vi "Autonomous.vi"   [LabVIEW 2017]
doc: "This VI starts when autonomous period begins, and will automatically be terminated when it ends. You can carry out timed or sensor driven operations directly to I/O or to subsystems without needing to return to the caller."
uses:
  <vilib>/Rock Robotics/WPI/Utilities/WPI_GetSetVariantRefNum.vi
  <vilib>/Rock Robotics/Network Tables/NT Read String.vi
types:
  T1 = typedef "WPI_JoystickDevRef.ctl" = cluster{"Device":T2}
  T2 = typedef "WPI_JoystickDeviceEnum.ctl" = enum16{"USB 0", "USB 1", "USB 2", "USB 3", "USB 4", "USB 5"}
  T3 = typedef "Command Status Info.ctl" = cluster{"Name":string, "Status":T4, "notifier out":T5}
  T4 = typedef "Completion Status.ctl" = enum16{"Successful", "Aborted", "Incomplete"}
  T5 = typedef "Completion Notifier.ctl" = refnum<notifier>
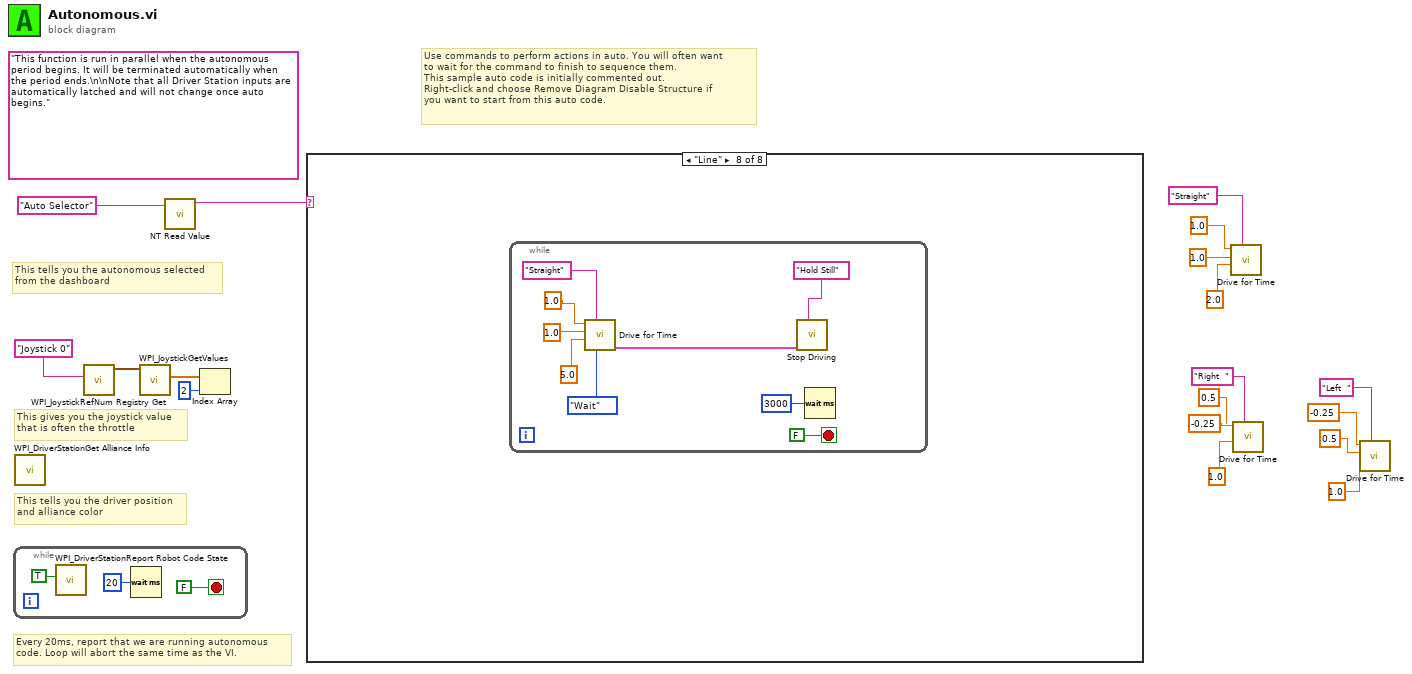
[diagram p0: block diagram]
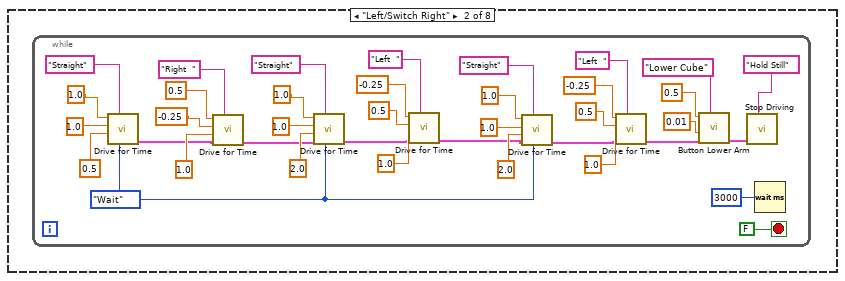
[diagram p3: hidden frame]
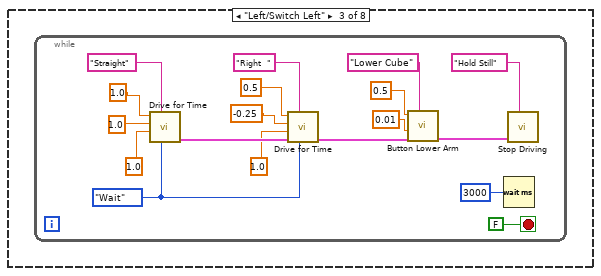
[diagram p4: hidden frame]
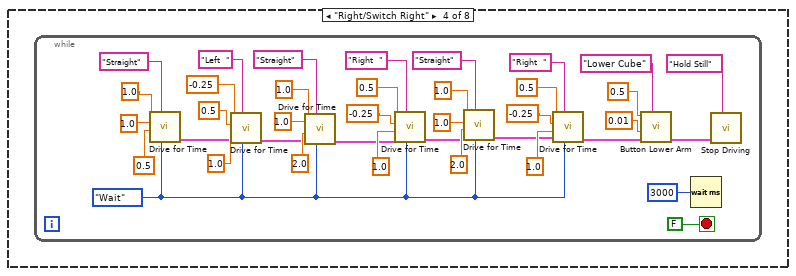
[diagram p5: hidden frame]
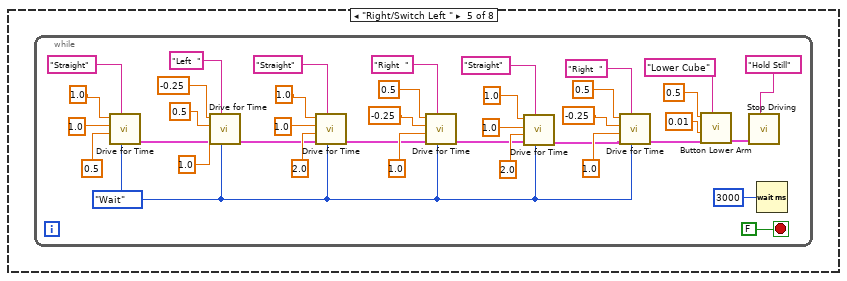
[diagram p6: hidden frame]
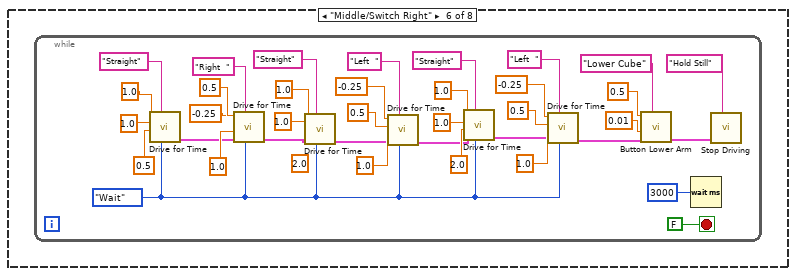
[diagram p7: hidden frame]
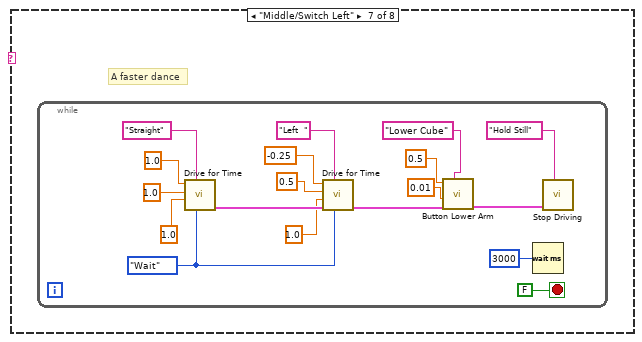
[diagram p8: hidden frame]
diagram:
  (unwired) "This function is run in parallel when the autonomous period begins. It will be terminated automatically when the period ends.\n\nNote that all Driver Station inputs are automatically latched and will not change once auto begins."
  # "Use commands to perform actions in auto. You will often want\nto wait for the command to finish to sequence them.\nThis sample auto code is initially commented out. \nRight-click and choose Remove Diagram Disable Structure if\nyou want to start from this auto code."
  # "This tells you the autonomous selected\nfrom the dashboard"
  # "Every 20ms, report that we are running autonomous\ncode. Loop will abort the same time as the VI."
  # "This gives you the joystick value\nthat is often the throttle"
  # "This tells you the driver position\nand alliance color"
  n1 = while {
    stop <- FALSE stop-if-true
    n2 = call <vilib>:"WPI_DriverStationReport Robot Code State.vi"("Autonomous"=TRUE) -> ()  [unwired: 10 in, 1 out]
    n3 = Wait (ms)(milliseconds to wait=u32 20) -> ()  [unwired: 1 out]
  }
  n4 = call <vilib>:"WPI_DriverStationGet Alliance Info.vi"() -> ()  [unwired: 12 out]
  n5 = call <vilib>:"WPI_JoystickRefNum Registry Get.vi"("refnum name"="Joystick 0") -> ("JoystickDevRef"=w17:T1)  [unwired: 1 in, 9 out]
  n6 = call <vilib>:"WPI_JoystickGetValues.vi"("JoystickDevRef"=w17) -> ("Axes"=w16:dbl[])  [unwired: 6 in, 4 out]
  n7 = call-poly <vilib>:"NT Read Value.vi"("Name"="Auto Selector") -> ("String"=w13:string)  [unwired: 9 in, 1 out]
  n8 = Index Array(array=w16, index=2) -> ()  [unwired: 1 out]
  n9 = case shown="\"Line\"" w13 {
    frame Default {
    }
    frame "Left/Switch Right" {
      n10 = while {
        stop <- FALSE stop-if-true
        w40 = enum16{"Start", "Wait"}."Wait" ("Synchronication")
        n11 = call "Drive for Time.vi"("Synchronization"=w40, "Description"="Straight", "Seconds"=0.5 ("Delay (s)"), "Right Speed"=1.0 ("X axis value"), "Left Speed"=1.0 ("X axis value")) -> ("Command Info Out"=w35:T3)  [unwired: 5 in, 1 out]
        n12 = call "Drive for Time.vi"("Description"="Right  ", "Command Info In"=w35, "Seconds"=1.0 ("Delay (s)"), "Right Speed"=-0.25 ("X axis value"), "Left Speed"=0.5 ("X axis value")) -> ("Command Info Out"=w34:T3)  [unwired: 5 in, 1 out]
        n13 = call "Drive for Time.vi"("Synchronization"=w40, "Description"="Straight", "Command Info In"=w34, "Seconds"=2.0 ("Delay (s)"), "Right Speed"=1.0 ("X axis value"), "Left Speed"=1.0 ("X axis value")) -> ("Command Info Out"=w29:T3)  [unwired: 4 in, 1 out]
        n14 = call "Drive for Time.vi"("Description"="Left  ", "Command Info In"=w29, "Seconds"=1.0 ("Delay (s)"), "Right Speed"=0.5 ("X axis value"), "Left Speed"=-0.25 ("X axis value")) -> ("Command Info Out"=w28:T3)  [unwired: 5 in, 1 out]
        n15 = call "Drive for Time.vi"("Synchronization"=w40, "Description"="Straight", "Command Info In"=w28, "Seconds"=2.0 ("Delay (s)"), "Right Speed"=1.0 ("X axis value"), "Left Speed"=1.0 ("X axis value")) -> ("Command Info Out"=w23:T3)  [unwired: 4 in, 1 out]
        n16 = call "Drive for Time.vi"("Description"="Left  ", "Command Info In"=w23, "Seconds"=1.0 ("Delay (s)"), "Right Speed"=0.5 ("X axis value"), "Left Speed"=-0.25 ("X axis value")) -> ("Command Info Out"=w22:T3)  [unwired: 5 in, 1 out]
        n17 = call "Button Lower Arm.vi"("Description"="Lower Cube", "Command Info In"=w22, "Deadband Value"=0.01, "Setpoint"=0.5) -> ("Command Info Out"=w57:T3)  [unwired: 7 in]
        n18 = call "Stop Driving.vi"("Description"="Hold Still", "Command Info In"=w57) -> ()  [unwired: 9 in, 1 out]
        n19 = Wait (ms)(milliseconds to wait=u32 3000 ("millisecond timer value")) -> ()  [unwired: 1 out]
      }
    }
    frame "Left/Switch Left" {
      n20 = while {
        stop <- FALSE stop-if-true
        w65 = enum16{"Start", "Wait"}."Wait" ("Synchronication")
        n21 = call "Drive for Time.vi"("Synchronization"=w65, "Description"="Straight", "Seconds"=1.0 ("Delay (s)"), "Right Speed"=1.0 ("X axis value"), "Left Speed"=1.0 ("X axis value")) -> ("Command Info Out"=w77:T3)  [unwired: 5 in, 1 out]
        n22 = call "Drive for Time.vi"("Synchronization"=w65, "Description"="Right  ", "Command Info In"=w77, "Seconds"=1.0 ("Delay (s)"), "Right Speed"=-0.25 ("X axis value"), "Left Speed"=0.5 ("X axis value")) -> ("Command Info Out"=w62:T3)  [unwired: 4 in, 1 out]
        n23 = call "Button Lower Arm.vi"("Description"="Lower Cube", "Command Info In"=w62, "Deadband Value"=0.01, "Setpoint"=0.5) -> ("Command Info Out"=w60:T3)  [unwired: 7 in]
        n24 = Wait (ms)(milliseconds to wait=u32 3000 ("millisecond timer value")) -> ()  [unwired: 1 out]
        n25 = call "Stop Driving.vi"("Description"="Hold Still", "Command Info In"=w60) -> ()  [unwired: 9 in, 1 out]
      }
    }
    frame "Right/Switch Right" {
      n26 = while {
        stop <- FALSE stop-if-true
        w78 = enum16{"Start", "Wait"}."Wait" ("Synchronication")
        n27 = call "Drive for Time.vi"("Synchronization"=w78, "Description"="Straight", "Seconds"=0.5 ("Delay (s)"), "Right Speed"=1.0 ("X axis value"), "Left Speed"=1.0 ("X axis value")) -> ("Command Info Out"=w95:T3)  [unwired: 5 in, 1 out]
        n28 = call "Drive for Time.vi"("Synchronization"=w78, "Description"="Left  ", "Command Info In"=w95, "Seconds"=1.0 ("Delay (s)"), "Right Speed"=0.5 ("X axis value"), "Left Speed"=-0.25 ("X axis value")) -> ("Command Info Out"=w90:T3)  [unwired: 4 in, 1 out]
        n29 = call "Drive for Time.vi"("Synchronization"=w78, "Description"="Straight", "Command Info In"=w90, "Seconds"=2.0 ("Delay (s)"), "Right Speed"=1.0 ("X axis value"), "Left Speed"=1.0 ("X axis value")) -> ("Command Info Out"=w85:T3)  [unwired: 4 in, 1 out]
        n30 = call "Drive for Time.vi"("Synchronization"=w78, "Description"="Right  ", "Command Info In"=w85, "Seconds"=1.0 ("Delay (s)"), "Right Speed"=-0.25 ("X axis value"), "Left Speed"=0.5 ("X axis value")) -> ("Command Info Out"=w80:T3)  [unwired: 4 in, 1 out]
        n31 = call "Drive for Time.vi"("Synchronization"=w78, "Description"="Straight", "Command Info In"=w80, "Seconds"=2.0 ("Delay (s)"), "Right Speed"=1.0 ("X axis value"), "Left Speed"=1.0 ("X axis value")) -> ("Command Info Out"=w79:T3)  [unwired: 4 in, 1 out]
        n32 = call "Drive for Time.vi"("Synchronization"=w78, "Description"="Right  ", "Command Info In"=w79, "Seconds"=1.0 ("Delay (s)"), "Right Speed"=-0.25 ("X axis value"), "Left Speed"=0.5 ("X axis value")) -> ("Command Info Out"=w102:T3)  [unwired: 4 in, 1 out]
        n33 = call "Button Lower Arm.vi"("Description"="Lower Cube", "Command Info In"=w102, "Deadband Value"=0.01, "Setpoint"=0.5) -> ("Command Info Out"=w100:T3)  [unwired: 7 in]
        n34 = Wait (ms)(milliseconds to wait=u32 3000 ("millisecond timer value")) -> ()  [unwired: 1 out]
        n35 = call "Stop Driving.vi"("Description"="Hold Still", "Command Info In"=w100) -> ()  [unwired: 9 in, 1 out]
      }
    }
    frame "Right/Switch Left " {
      n36 = while {
        stop <- FALSE stop-if-true
        w116 = enum16{"Start", "Wait"}."Wait" ("Synchronication")
        n37 = call "Drive for Time.vi"("Synchronization"=w116, "Description"="Straight", "Seconds"=0.5 ("Delay (s)"), "Right Speed"=1.0 ("X axis value"), "Left Speed"=1.0 ("X axis value")) -> ("Command Info Out"=w134:T3)  [unwired: 5 in, 1 out]
        n38 = call "Drive for Time.vi"("Synchronization"=w116, "Description"="Left  ", "Command Info In"=w134, "Seconds"=1.0 ("Delay (s)"), "Right Speed"=0.5 ("X axis value"), "Left Speed"=-0.25 ("X axis value")) -> ("Command Info Out"=w129:T3)  [unwired: 4 in, 1 out]
        n39 = call "Drive for Time.vi"("Synchronization"=w116, "Description"="Straight", "Command Info In"=w129, "Seconds"=2.0 ("Delay (s)"), "Right Speed"=1.0 ("X axis value"), "Left Speed"=1.0 ("X axis value")) -> ("Command Info Out"=w128:T3)  [unwired: 4 in, 1 out]
        n40 = call "Drive for Time.vi"("Synchronization"=w116, "Description"="Right  ", "Command Info In"=w128, "Seconds"=1.0 ("Delay (s)"), "Right Speed"=-0.25 ("X axis value"), "Left Speed"=0.5 ("X axis value")) -> ("Command Info Out"=w123:T3)  [unwired: 4 in, 1 out]
        n41 = call "Drive for Time.vi"("Synchronization"=w116, "Description"="Straight", "Command Info In"=w123, "Seconds"=2.0 ("Delay (s)"), "Right Speed"=1.0 ("X axis value"), "Left Speed"=1.0 ("X axis value")) -> ("Command Info Out"=w118:T3)  [unwired: 4 in, 1 out]
        n42 = call "Drive for Time.vi"("Synchronization"=w116, "Description"="Right  ", "Command Info In"=w118, "Seconds"=1.0 ("Delay (s)"), "Right Speed"=-0.25 ("X axis value"), "Left Speed"=0.5 ("X axis value")) -> ("Command Info Out"=w117:T3)  [unwired: 4 in, 1 out]
        n43 = call "Button Lower Arm.vi"("Description"="Lower Cube", "Command Info In"=w117, "Deadband Value"=0.01, "Setpoint"=0.5) -> ("Command Info Out"=w151:T3)  [unwired: 7 in]
        n44 = call "Stop Driving.vi"("Description"="Hold Still", "Command Info In"=w151) -> ()  [unwired: 9 in, 1 out]
        n45 = Wait (ms)(milliseconds to wait=u32 3000 ("millisecond timer value")) -> ()  [unwired: 1 out]
      }
    }
    frame "Middle/Switch Right" {
      n46 = while {
        stop <- FALSE stop-if-true
        (unwired) 2.0 ("Delay (s)")
        w154 = enum16{"Start", "Wait"}."Wait" ("Synchronication")
        n47 = call "Drive for Time.vi"("Synchronization"=w154, "Description"="Straight", "Seconds"=0.5 ("Delay (s)"), "Right Speed"=1.0 ("X axis value"), "Left Speed"=1.0 ("X axis value")) -> ("Command Info Out"=w160:T3)  [unwired: 5 in, 1 out]
        n48 = call "Drive for Time.vi"("Synchronization"=w154, "Description"="Right  ", "Command Info In"=w160, "Seconds"=1.0 ("Delay (s)"), "Right Speed"=-0.25 ("X axis value"), "Left Speed"=0.5 ("X axis value")) -> ("Command Info Out"=w159:T3)  [unwired: 4 in, 1 out]
        n49 = call "Drive for Time.vi"("Synchronization"=w154, "Description"="Straight", "Command Info In"=w159, "Right Speed"=1.0 ("X axis value"), "Left Speed"=1.0 ("X axis value")) -> ("Command Info Out"=w158:T3)  [unwired: 5 in, 1 out]
        n50 = call "Drive for Time.vi"("Synchronization"=w154, "Description"="Left  ", "Command Info In"=w158, "Seconds"=1.0 ("Delay (s)"), "Right Speed"=0.5 ("X axis value"), "Left Speed"=-0.25 ("X axis value")) -> ("Command Info Out"=w157:T3)  [unwired: 4 in, 1 out]
        n51 = call "Drive for Time.vi"("Synchronization"=w154, "Description"="Straight", "Command Info In"=w157, "Seconds"=2.0 ("Delay (s)"), "Right Speed"=1.0 ("X axis value"), "Left Speed"=1.0 ("X axis value")) -> ("Command Info Out"=w156:T3)  [unwired: 4 in, 1 out]
        n52 = call "Drive for Time.vi"("Synchronization"=w154, "Description"="Left  ", "Command Info In"=w156, "Seconds"=1.0 ("Delay (s)"), "Right Speed"=0.5 ("X axis value"), "Left Speed"=-0.25 ("X axis value")) -> ("Command Info Out"=w155:T3)  [unwired: 4 in, 1 out]
        n53 = call "Button Lower Arm.vi"("Description"="Lower Cube", "Command Info In"=w155, "Deadband Value"=0.01, "Setpoint"=0.5) -> ("Command Info Out"=w180:T3)  [unwired: 7 in]
        n54 = Wait (ms)(milliseconds to wait=u32 3000 ("millisecond timer value")) -> ()  [unwired: 1 out]
        n55 = call "Stop Driving.vi"("Description"="Hold Still", "Command Info In"=w180) -> ()  [unwired: 9 in, 1 out]
      }
    }
    frame "Middle/Switch Left" {
      # "A faster dance"
      n56 = while {
        stop <- FALSE stop-if-true
        w203 = enum16{"Start", "Wait"}."Wait" ("Synchronication")
        n57 = call "Drive for Time.vi"("Synchronization"=w203, "Description"="Straight", "Seconds"=1.0 ("Delay (s)"), "Right Speed"=1.0 ("X axis value"), "Left Speed"=1.0 ("X axis value")) -> ("Command Info Out"=w204:T3)  [unwired: 5 in, 1 out]
        n58 = call "Drive for Time.vi"("Synchronization"=w203, "Description"="Left  ", "Command Info In"=w204, "Seconds"=1.0 ("Delay (s)"), "Right Speed"=0.5 ("X axis value"), "Left Speed"=-0.25 ("X axis value")) -> ("Command Info Out"=w205:T3)  [unwired: 4 in, 1 out]
        n59 = call "Button Lower Arm.vi"("Description"="Lower Cube", "Command Info In"=w205, "Deadband Value"=0.01, "Setpoint"=0.5) -> ("Command Info Out"=w206:T3)  [unwired: 7 in]
        n60 = Wait (ms)(milliseconds to wait=u32 3000 ("millisecond timer value")) -> ()  [unwired: 1 out]
        n61 = call "Stop Driving.vi"("Description"="Hold Still", "Command Info In"=w206) -> ()  [unwired: 9 in, 1 out]
      }
    }
    frame "Line" {
      n62 = while {
        stop <- FALSE stop-if-true
        n63 = call "Drive for Time.vi"("Synchronization"=enum16{"Start", "Wait"}."Wait" ("Synchronication"), "Description"="Straight", "Seconds"=5.0 ("Delay (s)"), "Right Speed"=1.0 ("X axis value"), "Left Speed"=1.0 ("X axis value")) -> ("Command Info Out"=w209:T3)  [unwired: 5 in, 1 out]
        n64 = call "Stop Driving.vi"("Description"="Hold Still", "Command Info In"=w209) -> ()  [unwired: 9 in, 1 out]
        n65 = Wait (ms)(milliseconds to wait=u32 3000 ("millisecond timer value")) -> ()  [unwired: 1 out]
      }
    }
  }
  n66 = call "Drive for Time.vi"("Description"="Straight", "Seconds"=2.0 ("Delay (s)"), "Right Speed"=1.0 ("X axis value"), "Left Speed"=1.0 ("X axis value")) -> ()  [unwired: 6 in, 2 out]
  n67 = call "Drive for Time.vi"("Description"="Right  ", "Seconds"=1.0 ("Delay (s)"), "Right Speed"=-0.25 ("X axis value"), "Left Speed"=0.5 ("X axis value")) -> ()  [unwired: 6 in, 2 out]
  n68 = call "Drive for Time.vi"("Description"="Left  ", "Seconds"=1.0 ("Delay (s)"), "Right Speed"=0.5 ("X axis value"), "Left Speed"=-0.25 ("X axis value")) -> ()  [unwired: 6 in, 2 out]
